vi "vTab_9205_CHx1.vi"() -> ()   [LabVIEW 2022 SP3]
uses:
  <vilib>/Utility/sysdir.llb/System Directory Type.ctl
  <vilib>/express/express analysis/Spectral/Block/exnSpectralBlock spectral measurements peak poly.vi
  <vilib>/express/express analysis/Spectral/Block/exnSpectralBlock spectral measurements peak DDT.vi
  <vilib>/ErrorRing/Error Ring.xnode
  <vilib>/express/express analysis/Spectral/XNode/ExpressSpectralMeasurementsBlockNode.xnode
  <vilib>/Utility/config.llb/NI_LVConfig.lvlib
panel:
  in  "mv/g":dbl=152.0
  out "SVING":bool caption="存檔"
  in  "Open Folder":bool
  in  "Enable Saving":bool
  in  "Status":bool
  out "Time":timestamp format="%<%Y/%m/%d   %H:%M:%S>T"
  in  "Tab Control":enum32{"觸發訊號", "參數設定"}(tab)
  out "TD-P2P-Ch 1":dbl
  out "FFT-P2P-Ch 1":dbl
  out "CH1-X-FFT":dynamicdata(graph)
  out "CH1-X-Timedomain":dynamicdata(graph)
  in  "Lower Cut-Off (Hz)":dbl=100.0
  in  "DAQ Device (請選取 NI 9234 )":tag="cDAQ1Mod1"
  in  "ABORT":bool
  in  "Run":bool
  out "DAQ Stoped":bool
  out "DAQ Data":dynamicdata(graph)
  in  "PAUSE":bool
  out "DAQ Error":errorcluster
  out "DAQ (N)":i32
  out "Main (N)":i32
  out "Buffer in Queue":i32(slide) scale=0.0..100.0
  out "Processed":dynamicdata(graph)
  in  "Sample Rate":dbl=10000.0 format="%#_13g"
  in  "Samples to Read":i32=10000
  # "使用前請至 參數設置 設定"
  # "本頁畫面顯示為 觸發後訊號"
  # "FFT Filter by useing High-pass with Lower Cut-Off (Hz)"
  # "擷取卡設定"
  # "(系統開啟後修改無效)"
  # "軟體觸發設定"
  # "(修改即套用)"
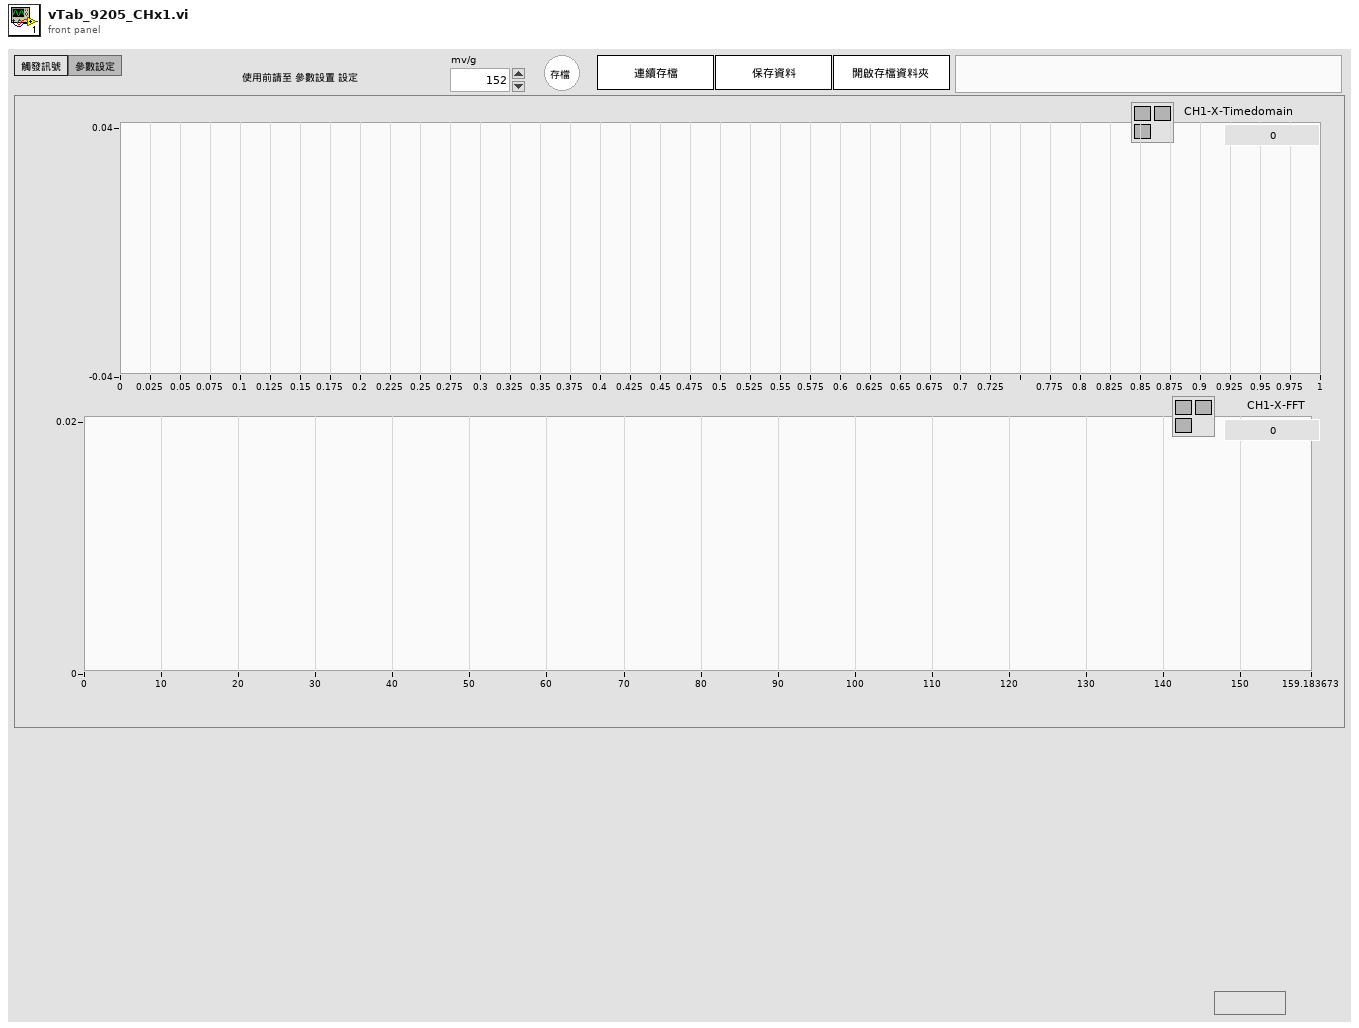
[diagram p1: front panel]
types:
  T1 = typedef "NI_LVConfig.lvlib/Config Data RefNum.ctl" = refnum<k1>
  T2 = enum8{"Enabled", "Disabled", "Disabled and Grayed Out"}
  T3 = cluster{"averaging mode":u16, "weighting mode":u16, "number of averages":u32}
  T4 = cluster{"dB On (F)":bool, "unwrap phase (F)":bool, "convert to degree (F)":bool}
  T5 = typedef "System Directory Type.ctl" = i32
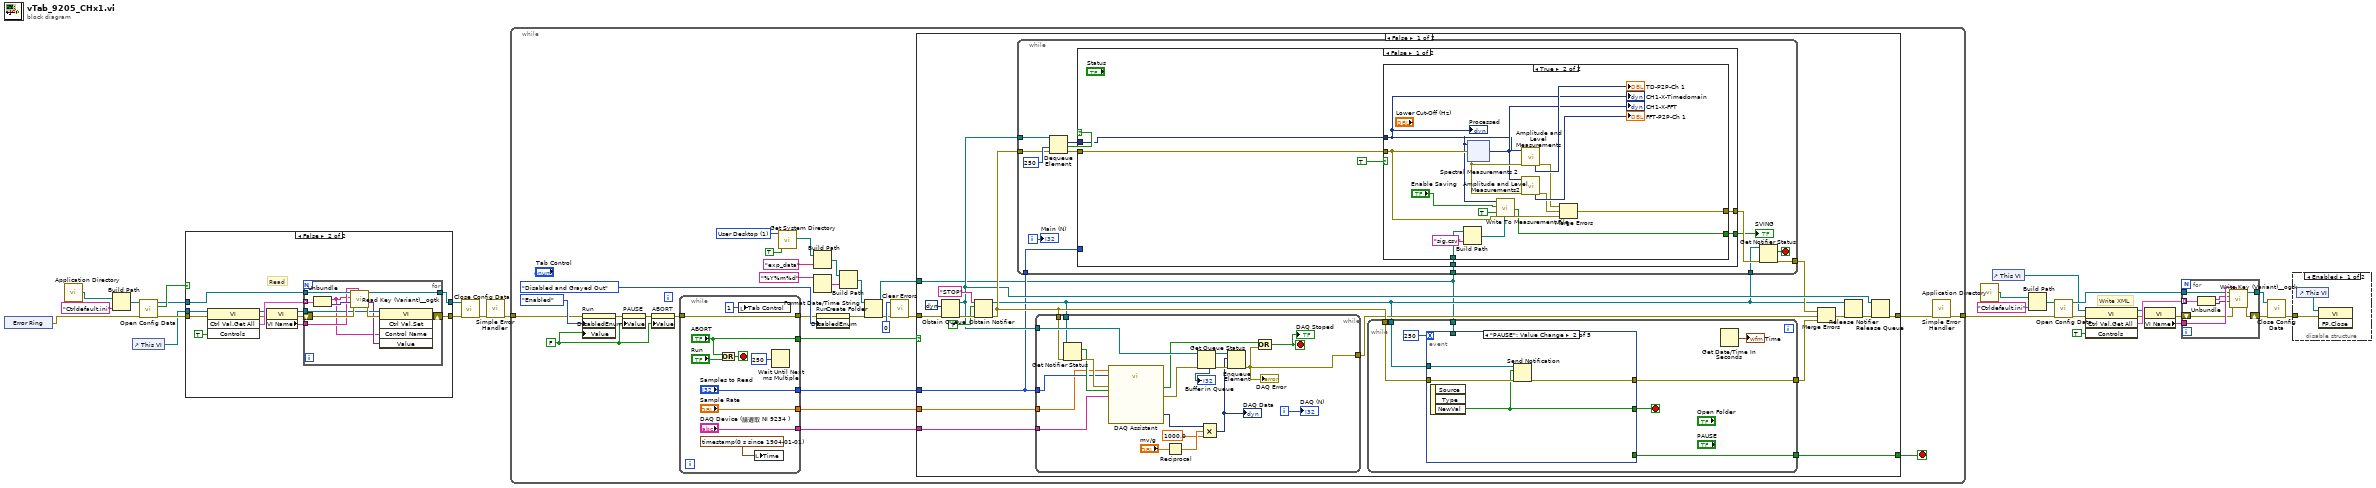
[diagram p0: block diagram]
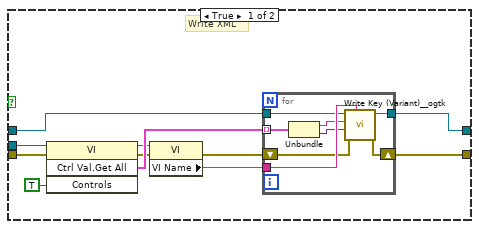
[diagram p2: hidden frame]
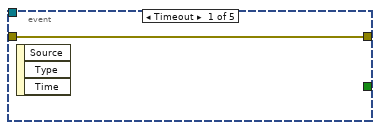
[diagram p6: hidden frame]
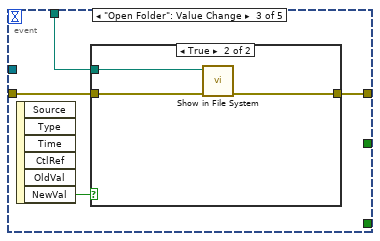
[diagram p7: hidden frame]
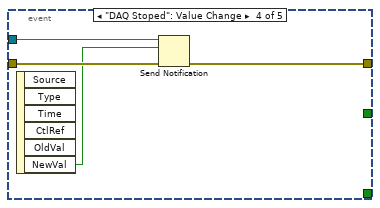
[diagram p9: hidden frame]
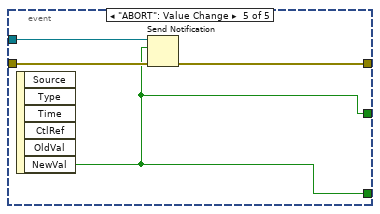
[diagram p10: hidden frame]
diagram:
  # "Write XML"
  n1 = xnode "Error Ring"() -> ("error out"=w20:errorcluster)
  n2 = call <vilib>:"Application Directory.vi"() -> ("Application Directory"=w1:path)
  n3 = Build Path(base path=w1, name or relative path="Ctrldefault.ini") -> (appended path=w28:path)
  n4 = control-ref of="This VI"() -> (w19:refnum<vi>)
  n5 = call <vilib>:"Open Config Data.vi"("error in (no error)"=w20, "configuration file path"=w28) -> ("error out"=w25:errorcluster, "file created?"=w21:bool, "refnum"=w18:T1)  [unwired: 7 in]
  n6 = case shown="False" w21 {
    tunnel: [w33 w53] -> w26
    tunnel: w25 -> [w31 w51]
    tunnel: [w29 w49] -> w24
    tunnel: w19 -> [w32 w52]
    tunnel: w18 -> [w34 w54]
    frame True {
      # "Write XML"
      n7 = invoke class="VI" method="Ctrl Val.Get All"(reference=w32, error in=w31, "Controls"=TRUE) -> (reference out=w38:refnum<vi>, error out=w37:errorcluster, "Get All Control Values Variant"=w39:cluster{"Name":string, "Variant Data":variant}[])  [unwired: 1 in, 1 out]
      n8 = property class="VI"(reference=w38, error in=w37) -> (error out=w30:errorcluster, "VI Name"=w36:string)  [unwired: 1 out]
      n9 = for {
        tunnel: w39 -> [w47] mode=indexing
        tunnel: w36 -> [w46]
        tunnel: w34 -> [w44]
        shift-right: [w43] -> w33
        shift-left: w30 -> [w41]
        tunnel: [w40] -> w29
        n10 = Unbundle(w47) -> ("Name"=w45:string, "Variant Data"=w42:variant)
        n11 = call <userlib>:"Write Key (Variant)__ogtk.vi"("section"=w46, "error in (no error)"=w41, "key-value"=w42, "key (optional)"=w45, "refnum"=w44) -> ("error out"=w43:errorcluster, "refnum out"=w40:T1)  [unwired: 5 in]
      }
    }
    frame False {
      # "Read"
      n12 = invoke class="VI" method="Ctrl Val.Get All"(reference=w52, error in=w51, "Controls"=TRUE) -> (reference out=w58:refnum<vi>, error out=w57:errorcluster, "Get All Control Values Variant"=w59:cluster{"Name":string, "Variant Data":variant}[])  [unwired: 1 in, 1 out]
      n13 = property class="VI"(reference=w58, error in=w57) -> (reference out=w48:refnum<vi>, error out=w50:errorcluster, "VI Name"=w56:string)
      n14 = for {
        tunnel: w59 -> [w70] mode=indexing
        tunnel: w56 -> [w63]
        tunnel: w54 -> [w69]
        shift-right: [w64] -> w53
        shift-left: w50 -> [w67]
        tunnel: [w66] -> w49
        tunnel: w48 -> [w62]
        n15 = Unbundle(w70) -> ("Name"=w60:string, "Variant Data"=w68:variant)
        n16 = call <userlib>:"Read Key (Variant)__ogtk.vi"("section"=w63, "error in (no error)"=w67, "type"=w68, "key (optional)"=w60, "refnum"=w69) -> ("error out"=w65:errorcluster, "key-value"=w61:variant, "refnum out"=w66:T1)  [unwired: 3 in, 1 out]
        n17 = invoke class="VI" method="Ctrl Val.Set"(reference=w62, error in=w65, "Control Name"=w60, "Value"=w61) -> (error out=w64:errorcluster)  [unwired: 1 in, 4 out]
      }
    }
  }
  n18 = call <vilib>:"Close Config Data.vi"("error in (no error)"=w26, "refnum"=w24) -> ("error out"=w23:errorcluster)  [unwired: 8 in, 1 out]
  n19 = call <vilib>:"Simple Error Handler.vi"("error in (no error)"=w23) -> ("error out"=w22:errorcluster)  [unwired: 4 in, 4 out]
  n20 = while {
    tunnel: [w98] -> w4
    tunnel: w22 -> [w73]
    stop <- w76 stop-if-true
    w87 = T5 1 items=["User Home"=0, "User Desktop"=1, "User Documents"=2, "User Application Data"=3, "User Preferences"=4, "User Temporary"=5, "Public Documents"=6, "Public Application Data"=7, "Public Preferences"=8, "Public Cache"=13, "System Core Libraries"=9, "System Installed Libraries"=10, "Application Files"=11, "Boot Volume Root"=12] ("system directory type")
    w92 = FALSE ("stop 3")
    n21 = property on="Run" class="Bool (strict)"(error in=w73, "DisabledEnum"=T2."Enabled" ("Disabled"), "Value"=w92) -> (error out=w95:errorcluster)  [unwired: 1 in, 1 out]
    n22 = property on="PAUSE" class="Bool (strict)"(error in=w95, "Value"=w92) -> (error out=w94:errorcluster)  [unwired: 1 in, 1 out]
    n23 = property on="ABORT" class="Bool (strict)"(error in=w94, "Value"=w92) -> (error out=w93:errorcluster)  [unwired: 1 in, 1 out]
    n24 = while {
      tunnel: [w227] -> w72
      tunnel: w93 -> [w227]
      tunnel: ["Samples to Read"] -> w75
      tunnel: ["Sample Rate"] -> w79
      tunnel: ["DAQ Device (請選取 NI 9234 )"] -> w77
      tunnel: ["ABORT"] -> w71
      stop <- w220 stop-if-true
      n25 = Or(x="ABORT", y="Run") -> (x .or. y?=w220:bool)
      n26 = local write "Tab Control"(1) -> ()
      n27 = local write "Time"(timestamp(0 s since 1904-01-01) ("Time 2")) -> ()
      n28 = Wait Until Next ms Multiple(millisecond multiple=u32 250) -> ()  [unwired: 1 out]
    }
    n29 = call <vilib>:"Get System Directory.vi"("create directory if not found? (F)"=TRUE, "system directory type"=w87) -> ("system directory"=w89:path)  [unwired: 9 in]
    n30 = Build Path(base path=w89, name or relative path="exp_data") -> (appended path=w85:path)
    n31 = Format Date/Time String(time format string (%c)="%Y%m%d") -> (date/time string=w84:string)  [unwired: 2 in]
    n32 = property on="Run" class="Bool (strict)"(error in=w72, "DisabledEnum"=T2."Disabled and Grayed Out" ("Disabled")) -> (error out=w90:errorcluster)  [unwired: 1 in, 1 out]
    n33 = Build Path(base path=w85, name or relative path=w84) -> (appended path=w83:path)
    n34 = Create Folder(path (use dialog)=w83, error in=w90) -> (created path=w74:path, error out=w81:errorcluster)  [unwired: 1 in, 1 out]
    n35 = call <vilib>:"Clear Errors.vi"("error in (no error)"=w81, "specific error code to clear (0: all)"=0) -> ("error out"=w80:errorcluster)  [unwired: 4 in, 1 out]
    n36 = case shown="False" w71 {
      selector: w71 -> [_ w216]
      tunnel: w80 -> [w110 w217]
      tunnel: w79 -> [w109 _]
      tunnel: [w106 w217] -> w78
      tunnel: w77 -> [w103 _]
      tunnel: [w101 w216] -> w76
      tunnel: w75 -> [w100 _]
      tunnel: w74 -> [w99 _]
      frame False {
        n37 = Obtain Queue(element data type=dynamicdata [] ("data"), error in (no error)=w110) -> (queue out=w108:refnum<queue>, error out=w113:errorcluster)  [unwired: 3 in, 1 out]
        n38 = Obtain Notifier(name (unnamed)="STOP", notification data type=FALSE, error in (no error)=w113) -> (notifier out=w102:refnum<notifier>, error out=w116:errorcluster)  [unwired: 1 in, 1 out]
        n39 = while {
          tunnel: w108 -> [w122]
          tunnel: w116 -> [w129]
          tunnel: [w125] -> w104
          tunnel: w102 -> [w123]
          tunnel: w100 -> [w120]
          tunnel: w99 -> [w119]
          i -> [w131]
          stop <- w124 stop-if-true
          n40 = Dequeue Element(queue=w122, timeout in ms (-1)=250, error in (no error)=w129) -> (element=w128:dynamicdata, timed out?=w121:bool, error out=w127:errorcluster)  [unwired: 1 out]
          n41 = case shown="False" w121 {
            tunnel: w128 -> [w136 _]
            tunnel: w127 -> [w135 w165]
            tunnel: [w137 w165] -> w126
            tunnel: w120 -> [_ _]
            tunnel: w119 -> [w133 _]
            tunnel: [w132 _] -> w118
            frame False {
              n42 = case shown="True" TRUE ("Data Available") {
                tunnel: w136 -> [_ w140]
                tunnel: w135 -> [w138 w141]
                tunnel: [w138 w148] -> w137
                tunnel: w133 -> [_ w145]
                tunnel: [_ w139] -> w132
                frame False {
                }
                frame True {
                  n43 = Build Path(base path=w145, name or relative path="sig.csv") -> (appended path=w143:path)
                  n44 = xnode ("Spectral Measurements 2")("Signals"=w140, "error in (no error)"=w141) -> ("FFT - (Peak)"=w142:dynamicdata, "error out"=w154:errorcluster)  [unwired: 1 out]
                  "CH1-X-FFT" <- w142
                  n45 = call "Write To Measurement File"("Signals"=w140, "Enable"="Enable Saving", "new_file"=TRUE, "error in (no error)"=w141, "Filename"=w143) -> ("Saving Data"=w139:bool, "error out"=w151:errorcluster)  [unwired: 12 in, 1 out]
                  n46 = call "Amplitude and Level Measurements"("Signals"=w140, "error in (no error)"=w154) -> ("Peak to Peak"=→"TD-P2P-Ch 1":dynamicdata, "error out"=w149:errorcluster)  [unwired: 12 out]
                  n47 = call "Amplitude and Level Measurements2"("Signals"=w142, "error in (no error)"=w154) -> ("Peak to Peak"=→"FFT-P2P-Ch 1":dynamicdata, "error out"=w150:errorcluster)  [unwired: 12 out]
                  n48 = Merge Errors(w149, w150, w151) -> (w148:errorcluster)
                  "Processed" <- w140
                  "CH1-X-Timedomain" <- w140
                }
              }
            }
            frame True {
            }
          }
          "SVING" <- w118
          n49 = Get Notifier Status(notifier=w123, error in (no error)=w126) -> (current notification=w124:bool, error out=w125:errorcluster)  [unwired: 3 out]
          "Main (N)" <- w131
        }
        n50 = while {
          tunnel: w108 -> [w184]
          tunnel: [w176] -> w115
          tunnel: w116 -> [w180]
          tunnel: w102 -> [w178]
          tunnel: w100 -> [w172]
          tunnel: w109 -> [w171]
          tunnel: w103 -> [w173]
          i -> [w186]
          stop <- w177 stop-if-true
          n51 = Get Notifier Status(notifier=w178, error in (no error)=w180) -> (current notification=w175:bool, error out=w179:errorcluster)  [unwired: 3 out]
          n52 = call "DAQ Assistant"("rate"=w171, "number of samples"=w172, "error in"=w179, "stop (F)"=w175, "device name"=w173) -> ("data"=w170:dynamicdata, "stopped"=w174:bool, "error out"=w181:errorcluster)  [unwired: 11 in, 1 out]
          n53 = Reciprocal(x="mv/g") -> (1/x=w167:dbl)
          n54 = Get Queue Status(queue=w184, error in (no error)=w181) -> (queue out=w183:refnum<queue>, error out=w182:errorcluster, # elements in queue=→"Buffer in Queue":i32)  [unwired: 1 in, 5 out]
          n55 = Compound Arithmetic op=MULTIPLY(w170, w167, 1000.0 ("value")) -> (w169:dynamicdata)
          "DAQ Data" <- w169
          n56 = Enqueue Element(queue=w183, element=w169, error in (no error)=w182) -> (error out=w176:errorcluster)  [unwired: 1 in, 2 out]
          "DAQ Error" <- w176
          n57 = Compound Arithmetic op=OR(w174, w176) -> (w177:bool)
          "DAQ Stoped" <- w177
          "DAQ (N)" <- w186
        }
        n58 = while {
          tunnel: w116 -> [w194]
          tunnel: [w193] -> w117
          tunnel: w102 -> [w191]
          tunnel: [w188] -> w101
          tunnel: w99 -> [w187]
          stop <- w189 stop-if-true
          n59 = event shown="[1] \"PAUSE\": Value Change" {
            selector: _ -> [_ _ _ _ _]
            dyn-events: _ -> [_ _ _ _ _]
            timeout: 250 -> [_ _ _ _ _]
            tunnel: w194 -> [w195 w199 w202 w211 w215]
            tunnel: [w195 w198 w200 w208 w214] -> w193
            tunnel: w191 -> [_ w197 _ w209 w213]
            tunnel: [_ w196 _ _ w212] -> w189
            tunnel: [_ _ _ _ w212] -> w188
            tunnel: w187 -> [_ _ w201 _ _]
            event Timeout {
              n60 = event-data() -> ()  [unwired: 1 in, 3 out]
            }
            event "PAUSE": Value Change {
              n61 = event-data() -> ("NewVal"=w196:bool)  [unwired: 1 in, 2 out]
              n62 = Send Notification(notification=w196, notifier=w197, error in (no error)=w199) -> (error out=w198:errorcluster)  [unwired: 1 out]
            }
            event "Open Folder": Value Change {
              n63 = event-data() -> ("NewVal"=w203:bool)  [unwired: 1 in, 5 out]
              n64 = case shown="True" w203 {
                tunnel: w202 -> [w204 w207]
                tunnel: w201 -> [_ w206]
                tunnel: [w204 w205] -> w200
                frame False {
                }
                frame True {
                  n65 = call <vilib>:"Show in File System.vi"("error in (no error)"=w207, "file or directory path"=w206) -> ("error out"=w205:errorcluster)  [unwired: 9 in]
                }
              }
            }
            event "DAQ Stoped": Value Change {
              n66 = event-data() -> ("NewVal"=w210:bool)  [unwired: 1 in, 5 out]
              n67 = Send Notification(notification=w210, notifier=w209, error in (no error)=w211) -> (error out=w208:errorcluster)  [unwired: 1 out]
            }
            event "ABORT": Value Change {
              n68 = event-data() -> ("NewVal"=w212:bool)  [unwired: 1 in, 5 out]
              n69 = Send Notification(notification=w212, notifier=w213, error in (no error)=w215) -> (error out=w214:errorcluster)  [unwired: 1 out]
            }
          }
          n70 = Get Date/Time In Seconds() -> (seconds since 1Jan1904=→"Time":timestamp)
        }
        n71 = Merge Errors(w104, w115, w117) -> (w105:errorcluster)
        n72 = Release Notifier(notifier=w102, error in (no error)=w105) -> (error out=w107:errorcluster)  [unwired: 1 in, 2 out]
        n73 = Release Queue(queue=w108, error in (no error)=w107) -> (error out=w106:errorcluster)  [unwired: 1 in, 2 out]
      }
      frame True {
      }
    }
    n74 = call <vilib>:"Simple Error Handler.vi"("error in (no error)"=w78) -> ("error out"=w98:errorcluster)  [unwired: 4 in, 4 out]
  }
  n75 = call <vilib>:"Application Directory.vi"() -> ("Application Directory"=w2:path)
  n76 = control-ref of="This VI"() -> (w16:refnum<vi>)
  n77 = Build Path(base path=w2, name or relative path="Ctrldefault.ini") -> (appended path=w11:path)
  n78 = call <vilib>:"Open Config Data.vi"("error in (no error)"=w4, "configuration file path"=w11) -> ("error out"=w14:errorcluster, "refnum"=w17:T1)  [unwired: 7 in, 1 out]
  n79 = invoke class="VI" method="Ctrl Val.Get All"(reference=w16, error in=w14, "Controls"=TRUE) -> (reference out=w9:refnum<vi>, error out=w8:errorcluster, "Get All Control Values Variant"=w10:cluster{"Name":string, "Variant Data":variant}[])  [unwired: 1 in, 1 out]
  n80 = property class="VI"(reference=w9, error in=w8) -> (error out=w5:errorcluster, "VI Name"=w7:string)  [unwired: 1 out]
  n81 = for {
    tunnel: w10 -> [w235] mode=indexing
    tunnel: w7 -> [w234]
    tunnel: w17 -> [w232]
    shift-right: [w231] -> w13
    shift-left: w5 -> [w229]
    tunnel: [w228] -> w15
    n82 = Unbundle(w235) -> ("Name"=w233:string, "Variant Data"=w230:variant)
    n83 = call <userlib>:"Write Key (Variant)__ogtk.vi"("section"=w234, "error in (no error)"=w229, "key-value"=w230, "key (optional)"=w233, "refnum"=w232) -> ("error out"=w231:errorcluster, "refnum out"=w228:T1)  [unwired: 5 in]
  }
  n84 = call <vilib>:"Close Config Data.vi"("error in (no error)"=w13, "refnum"=w15) -> ("error out"=w3:errorcluster)  [unwired: 8 in, 1 out]
  n85 = disable-structure shown="Enabled" {
    disable-tunnel: w3 -> [w236 _]
    frame Enabled {
      n86 = control-ref of="This VI"() -> (w237:refnum<vi>)
      n87 = invoke class="VI" method="FP.Close"(reference=w237, error in=w236) -> ()  [unwired: 1 in, 3 out]
    }
    frame Disabled {
    }
  }
